vi "ExperimentCodeUpdateLoop.vi"(8 "milliseconds to wait":u32=100, 9 "EventData in":refnum<user-event>, 10 "MEditor":refnum<k24>, 11 "ExperimentID":refnum<vi>) -> ()   [LabVIEW 2017]
uses:
  C:/Code/CMCryoSysCode/CSharp/MatlabEditor/MatlabEditor/bin/Debug/MatlabEditor.dll
  CSharp/MatlabEditor/MatlabEditor/bin/Debug/MatlabEditor.dll
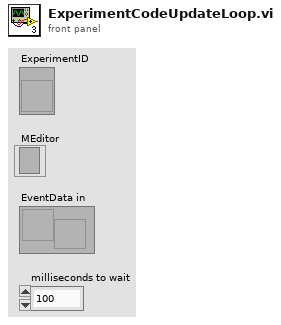
[diagram p1: front panel]
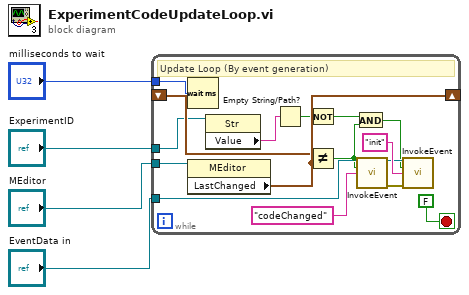
[diagram p0: block diagram]
diagram:
  n1 = while {
    tunnel: "EventData in" -> [w14]
    tunnel: "MEditor" -> [w18]
    shift-right: [w17] -> _
    shift-left: _ -> [w16]
    tunnel: "ExperimentID" -> [w7]
    tunnel: "milliseconds to wait" -> [w6]
    stop <- FALSE stop-if-true
    # "Update Loop (By event generation)"
    n2 = Wait (ms)(milliseconds to wait=w6) -> ()  [unwired: 1 out]
    n3 = property class="MEditor"(reference=w18) -> ("LastChanged"=w17:timestamp)  [unwired: 1 in, 2 out]
    n4 = property class="Str"(reference=w7) -> ("Value"=w5:string)  [unwired: 1 in, 2 out]
    n5 = Empty String/Path?(string/path=w5) -> (empty?=w9:bool)
    n6 = Not(x=w9) -> (.not. x?=w8:bool)
    n7 = Not Equal?(x=w16, y=w17) -> (x != y?=w11:bool)
    n8 = And(x=w8, y=w11) -> (x .and. y?=w10:bool)
    n9 = call "InvokeEvent.vi"("Event Stream In"=w14, "Invoke?"=w11, "name"="codeChanged") -> ("Event Stream Out"=w12:refnum<user-event>, "error out"=w13:errorcluster)  [unwired: 11 in]
    n10 = call "InvokeEvent.vi"("Event Stream In"=w12, "Invoke?"=w10, "name"="init", "error in (no error)"=w13) -> ()  [unwired: 10 in, 2 out]
  }
